vi "Write AO Voltage.vi"(8 "error in (no error)":errorcluster caption="错误输入（无错误）", 10 "data":dbl caption="数据" format="%0.2f", 11 "DAQ 输入":refnum<class "DAQ.lvclass">) -> (0 "error out":errorcluster caption="错误输出", 3 "DAQ 输出":refnum<class "DAQ.lvclass">)   [LabVIEW 2017, in "DAQ.lvlib" / "DAQ.lvclass"]
uses:
  DAQ.lvclass
  E:/Program Files (x86)/National Instruments/LabVIEW 2017/vi.lib/ActorFramework/Actor/Actor.lvclass
  <vilib>/ActorFramework/Actor/Actor.lvclass/Actor.ctl
  DAQ.lvclass/DAQ.ctl
  <vilib>/ActorFramework/Message Enqueuer/Message Enqueuer.lvclass/Message Enqueuer.ctl
  <vilib>/DAQmx/write.llb/DAQmx Write (Analog DBL 1Chan 1Samp).vi
  <vilib>/ActorFramework/Message Enqueuer/Enqueue.vi
  E:/Program Files (x86)/National Instruments/LabVIEW 2017/vi.lib/ActorFramework/Message/Message.lvclass
  <vilib>/ActorFramework/Message Priority Queue/Priority Enqueue.vi
  <vilib>/DAQmx/create/channels.llb/DAQmx Create Channel (AO-Voltage-Basic).vi
  <vilib>/DAQmx/miscellaneous.llb/DAQmx Fill In Error Info.vi
  <vilib>/ActorFramework/Actor/Actor.lvclass
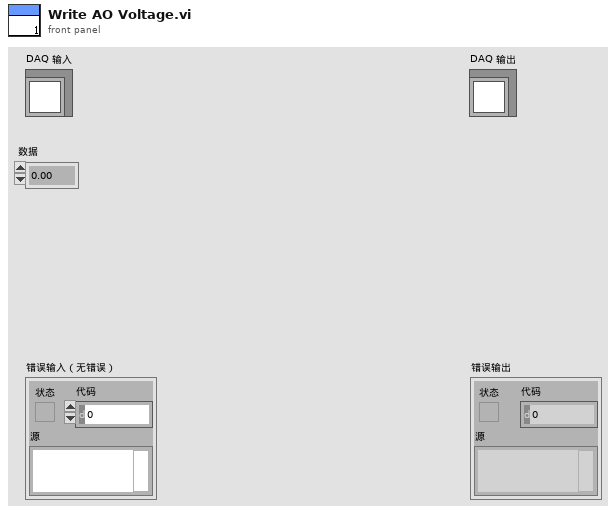
[diagram p1: front panel]
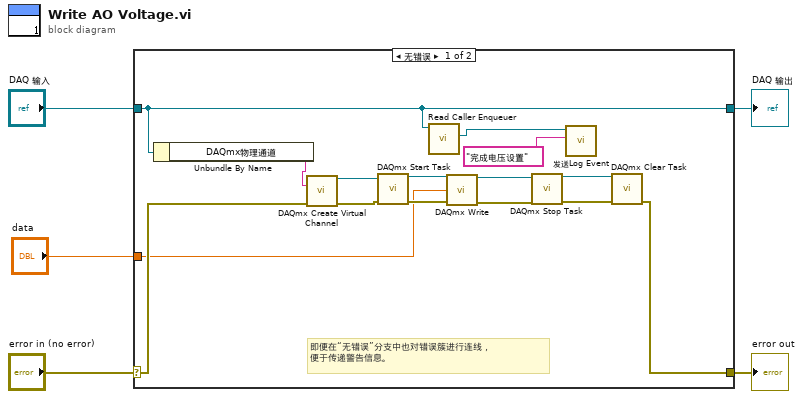
[diagram p0: block diagram]
diagram:
  n1 = case shown="无错误" "error in (no error)" {
    selector: "error in (no error)" -> [w20 w22]
    tunnel: [w11 w22] -> w4
    tunnel: [w8 w21] -> w2
    tunnel: "DAQ 输入" -> [w8 w21]
    tunnel: "data" -> [w9 _]
    frame No Error {
      # "即便在“无错误”分支中也对错误簇进行连线，\n便于传递警告信息。"
      n2 = Unbundle By Name(w8) -> ("DAQmx物理通道"=w10:tag)
      n3 = call-poly <vilib>:"DAQmx Create Virtual Channel.vi"("physical channels"=w10, "error in"=w20) -> ("task out"=w18:refnum<k21>, "error out"=w19:errorcluster)  [unwired: 12 in]
      n4 = call <vilib>:"DAQmx Start Task.vi"("task/channels in"=w18, "error in"=w19) -> ("task out"=w17:refnum<k21>, "error out"=w16:errorcluster)  [unwired: 12 in]
      n5 = call <vilib>:"Read Caller Enqueuer.vi"("Actor"=w8) -> ("Caller Enqueuer"=w7:refnum<class "Message Enqueuer.lvclass">)  [unwired: 10 in]
      n6 = call-poly <vilib>:"DAQmx Write.vi"("task/channels in"=w17, "data"=w9, "error in"=w16) -> ("task out"=w14:refnum<k21>, "error out"=w15:errorcluster)  [unwired: 10 in, 1 out]
      n7 = call <vilib>:"DAQmx Stop Task.vi"("task/channels in"=w14, "error in"=w15) -> ("task out"=w12:refnum<k21>, "error out"=w13:errorcluster)  [unwired: 12 in]
      n8 = call "发送Log Event.vi"("事件文本"="完成电压设置", "Message Enqueuer"=w7) -> ()  [unwired: 8 in, 2 out]
      n9 = call <vilib>:"DAQmx Clear Task.vi"("task in"=w12, "error in"=w13) -> ("error out"=w11:errorcluster)  [unwired: 13 in]
    }
    frame Error {
    }
  }
  "error out" <- w4
  "DAQ 输出" <- w2
